vi "Leaderboard test 5.vi"(11 "current time":timestamp) -> ()   [LabVIEW 2020, in "Visualisation.lvclass"]
uses:
  Visualisation.lvclass
  Application/Globals.vi
  Data Manager/Data Manager.lvclass
  Application/Application.lvlib
panel:
  out "Daily Change B":dbl format="+ %0.1f km"
  out "Daily Change A":dbl format="+ %0.1f km"
  out "Table Control":string[][](table)
  out "Line 3":string
  out "Group Totals 6":dbl format="%0.1f km"
  out "Group Totals 5":dbl format="%0.1f km"
  out "Line 2":string
  out "Group Totals 4":dbl format="%0.1f km"
  out "Group Totals 3":dbl format="%0.1f km"
  out "Line 1":string
  out "Group Totals 2":dbl format="%0.1f km"
  out "Group Totals 1":dbl format="%0.1f km"
  out "Walk":T1(array[cluster]) {"Distance 2" scale=0.0..92.6965}
  out "Leaderboard":T2(array[cluster]) {"Distance" scale=0.0..167.7288}
  out "Ride":T3(array[cluster]) {"Distance 4" scale=0.0..76.5197}
  out "Run":T1(array[cluster]) {"Distance 2" scale=0.0..96.2213}
  out "B Total":dbl format="%0.1f km"
  out "A Total":dbl format="%0.1f km"
  # "Total Distance Leaderboard"
  # "Head to Head"
  # "VS"
  # "VS"
  # "VS"
  # "Longest Single Activity"
  # "Daily Total Distance Change"
  # "VS"
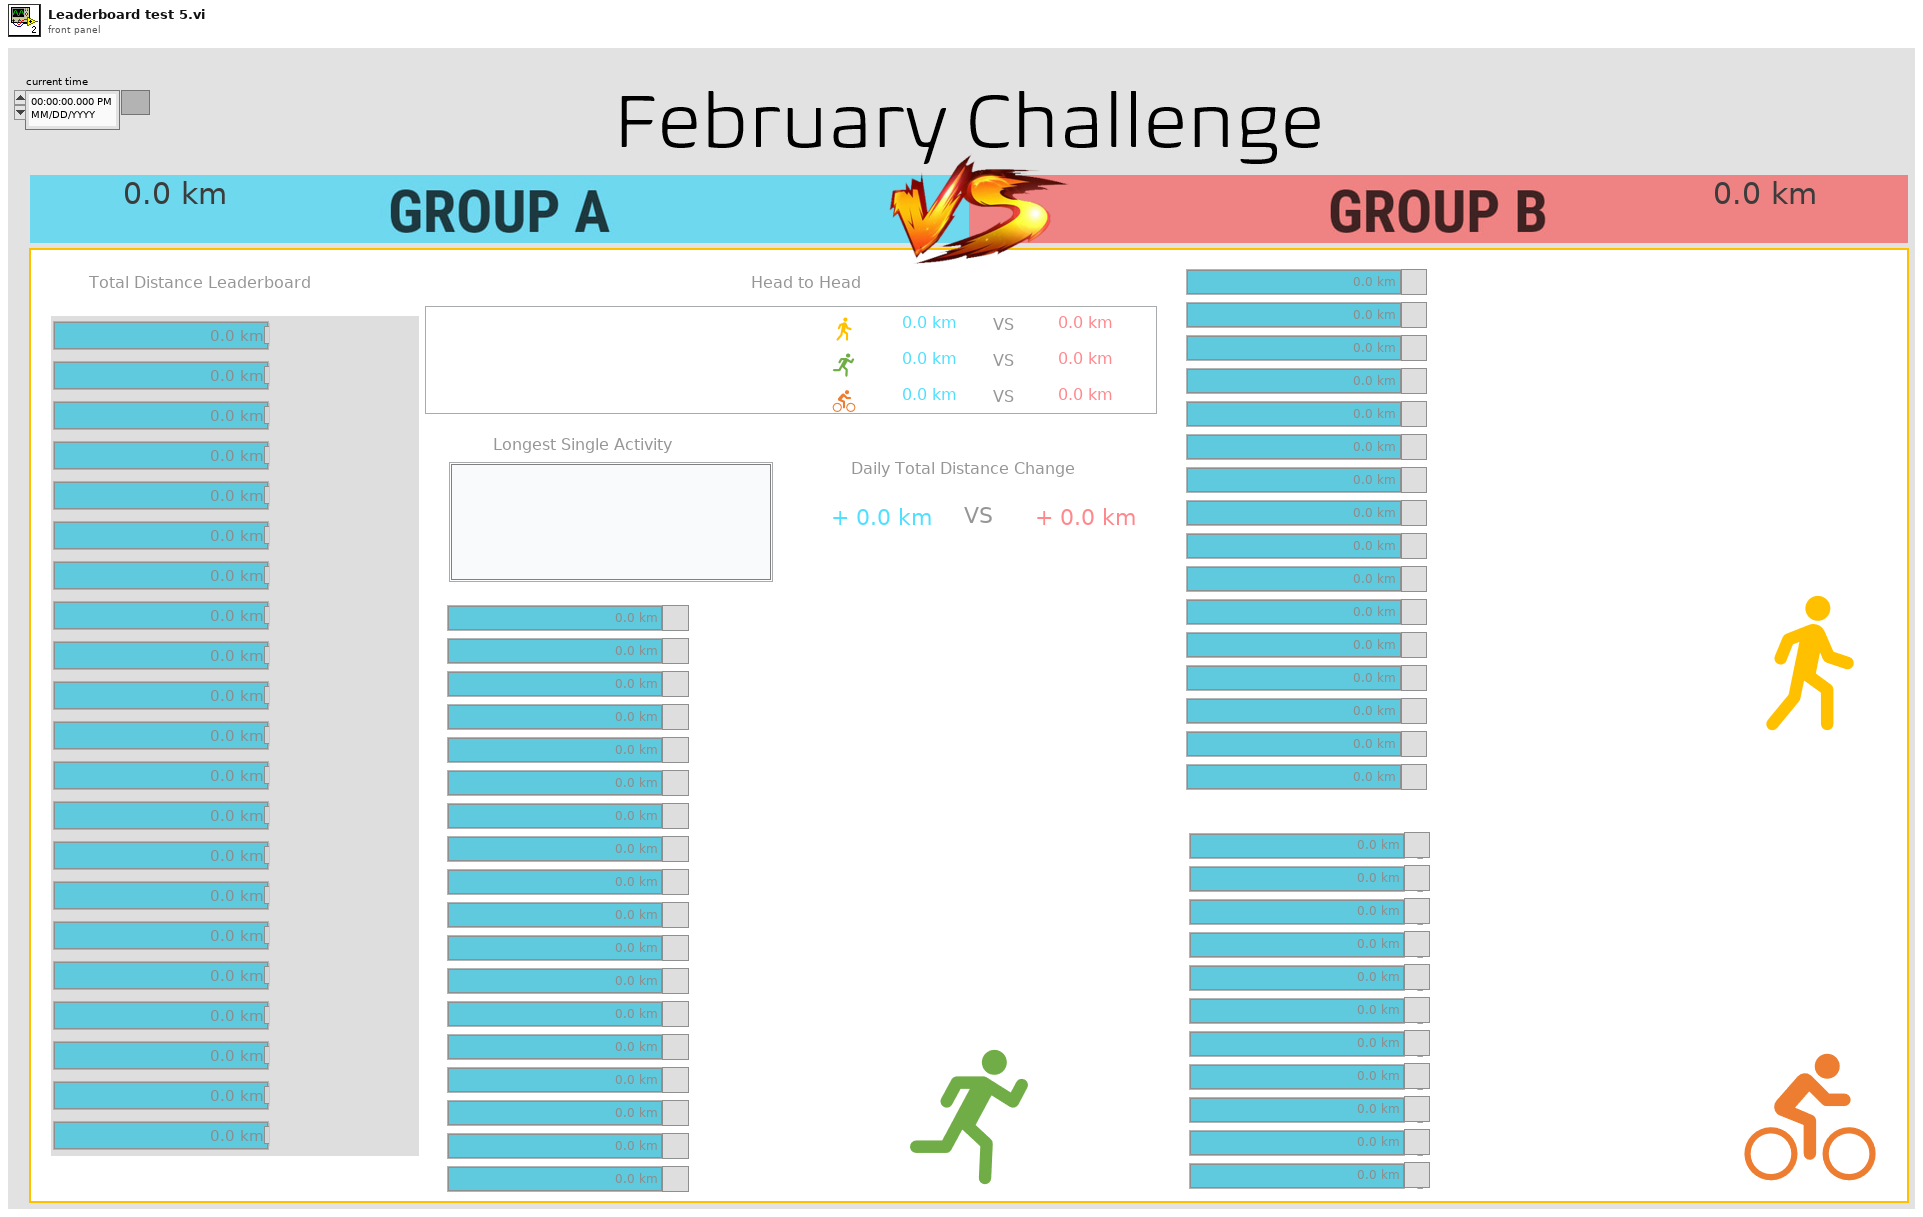
[diagram p1: front panel]
types:
  T1 = cluster{"Athlete":string, "Team":u32, "Distance 2":dbl}[]
  T2 = cluster{"Athlete":string, "Distance":dbl, "Team":u32}[]
  T3 = cluster{"Athlete":string, "Team":u32, "Distance 4":dbl}[]
  T4 = cluster{"Athlete":string, "Team":u32, "Distance 2":dbl}
  T5 = cluster{"Athlete":string, "Distance":dbl, "Team":u32, "Distance 2":cluster{"Numeric":dbl, "Numeric":dbl, "Numeric":dbl}}
  T6 = cluster{"Athlete":string, "Distance":dbl, "Team":u32}
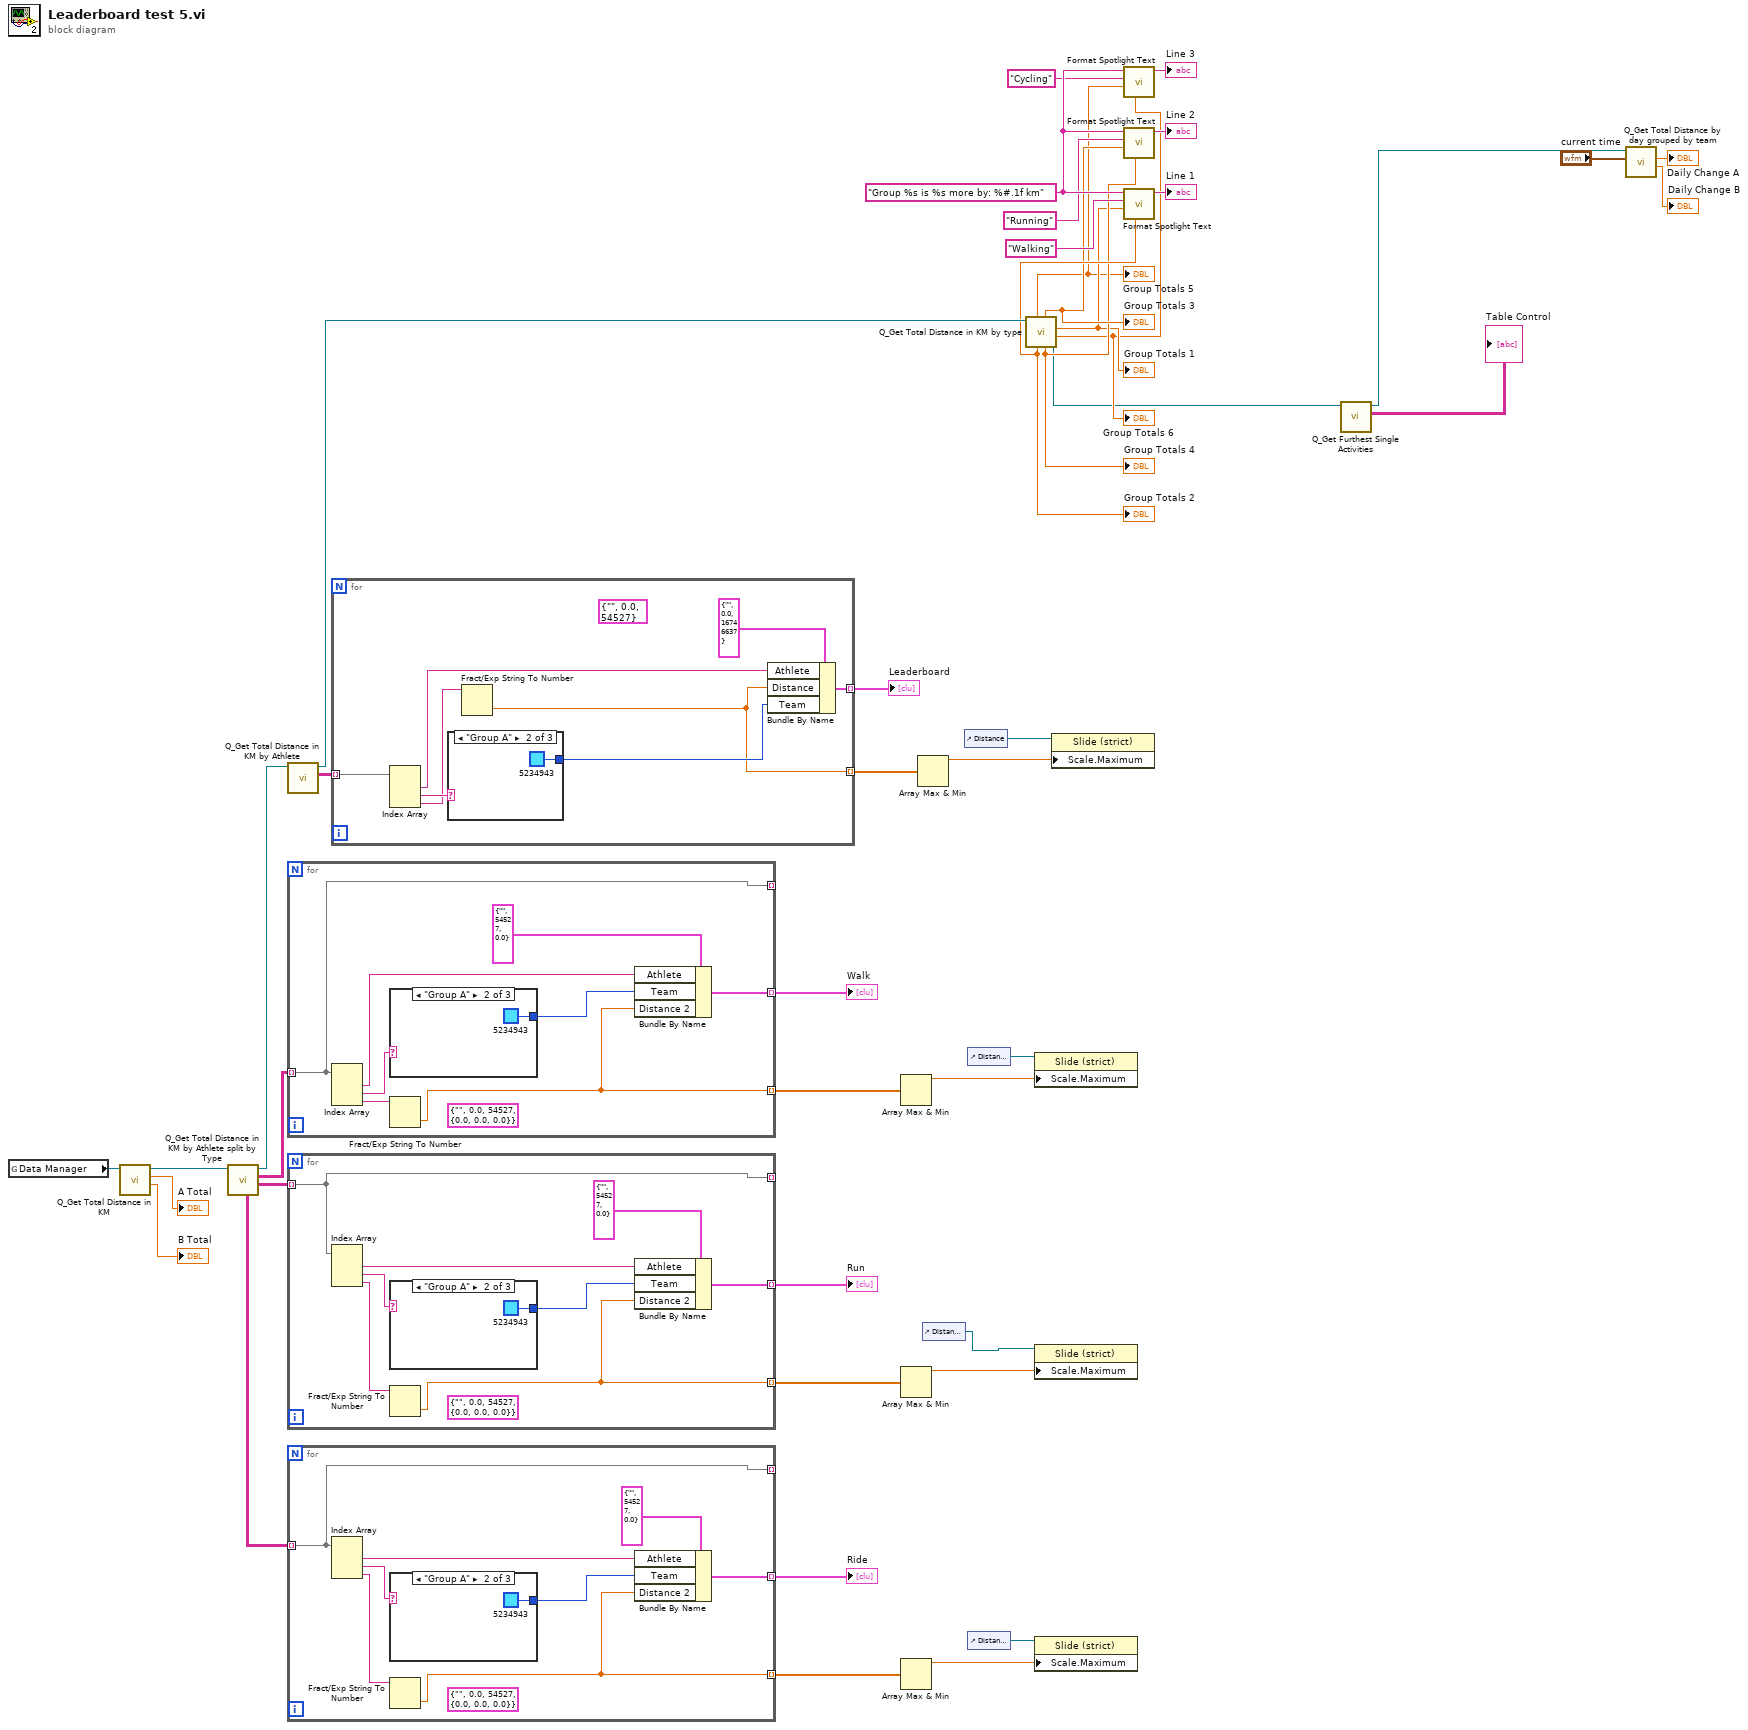
[diagram p0: block diagram]
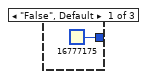
[diagram p2: hidden frame]
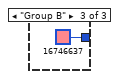
[diagram p3: hidden frame]
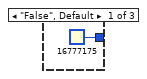
[diagram p4: hidden frame]
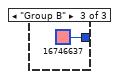
[diagram p5: hidden frame]
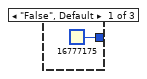
[diagram p6: hidden frame]
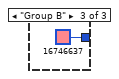
[diagram p7: hidden frame]
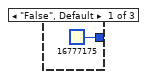
[diagram p8: hidden frame]
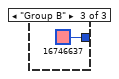
[diagram p9: hidden frame]
diagram:
  w16 = "Group %s is %s more by: %#.1f km"
  n1 = global read "Globals.vi" "Data Manager"() -> (w45:refnum<class "Data Manager.lvclass">)
  n2 = call-dynamic "Q_Get Total Distance in KM.vi"("Data Manager in"=w45) -> ("Group B"=→"B Total":dbl, "Group A"=→"A Total":dbl, "Data Manager out"=w40:refnum<class "Data Manager.lvclass">)  [unwired: 6 in, 2 out]
  n3 = call-dynamic "Q_Get Total Distance in KM by Athlete split by Type.vi"("Data Manager in"=w40) -> ("Run"=w35:string[][], "Walk"=w39:string[][], "Data Manager out"=w28:refnum<class "Data Manager.lvclass">, "Ride"=w32:string[][])  [unwired: 6 in, 1 out]
  n4 = call-dynamic "Q_Get Total Distance in KM by Athlete.vi"("Data Manager in"=w28) -> ("Result Set"=w27:string[][], "Data Manager out"=w20:refnum<class "Data Manager.lvclass">)  [unwired: 8 in, 1 out]
  n5 = for {
    tunnel: [w48] -> _ mode=indexing
    tunnel: [w53] -> w22 mode=indexing
    tunnel: w39 -> [w48] mode=indexing
    tunnel: [w47] -> w36 mode=indexing
    (unwired) T5 {"Athlete"="", "Distance"=0.0, "Team"=54527, "Distance 2"={"Numeric"=0.0, "Numeric"=0.0, "Numeric"=0.0}} ("Leaderboard")
    n6 = Index Array(array=w48) -> (element #1=w49:string, element #2=w51:string, element #3=w50:string)  [unwired: 3 in]
    n7 = case shown="\"Group A\"" w51 {
      tunnel: [u32 16777175 ("Color Box") u32 5234943 ("Color Box") u32 16746637 ("Color Box")] -> w52
      frame "False", Default {
      }
      frame "Group A" {
      }
      frame "Group B" {
      }
    }
    n8 = Fract/Exp String To Number(string=w50) -> (number=w47:dbl)  [unwired: 3 in, 1 out]
    n9 = Bundle By Name(cluster=T4 {"Athlete"="", "Team"=54527, "Distance 2"=0.0} ("Leaderboard"), "Athlete"=w49, "Team"=w52, "Distance 2"=w47) -> (w53:T4)
  }
  "Walk" <- w22
  n10 = for {
    tunnel: w35 -> [w59] mode=indexing
    tunnel: [w64] -> w33 mode=indexing
    tunnel: [w59] -> _ mode=indexing
    tunnel: [w58] -> w34 mode=indexing
    (unwired) T5 {"Athlete"="", "Distance"=0.0, "Team"=54527, "Distance 2"={"Numeric"=0.0, "Numeric"=0.0, "Numeric"=0.0}} ("Leaderboard")
    n11 = Index Array(array=w59) -> (element #1=w60:string, element #2=w62:string, element #3=w61:string)  [unwired: 3 in]
    n12 = case shown="\"Group A\"" w62 {
      tunnel: [u32 16777175 ("Color Box") u32 5234943 ("Color Box") u32 16746637 ("Color Box")] -> w63
      frame "False", Default {
      }
      frame "Group A" {
      }
      frame "Group B" {
      }
    }
    n13 = Fract/Exp String To Number(string=w61) -> (number=w58:dbl)  [unwired: 3 in, 1 out]
    n14 = Bundle By Name(cluster=T4 {"Athlete"="", "Team"=54527, "Distance 2"=0.0} ("Leaderboard"), "Athlete"=w60, "Team"=w63, "Distance 2"=w58) -> (w64:T4)
  }
  "Run" <- w33
  n15 = for {
    tunnel: w32 -> [w70] mode=indexing
    tunnel: [w75] -> w30 mode=indexing
    tunnel: [w70] -> _ mode=indexing
    tunnel: [w69] -> w31 mode=indexing
    (unwired) T5 {"Athlete"="", "Distance"=0.0, "Team"=54527, "Distance 2"={"Numeric"=0.0, "Numeric"=0.0, "Numeric"=0.0}} ("Leaderboard")
    n16 = Index Array(array=w70) -> (element #1=w71:string, element #2=w73:string, element #3=w72:string)  [unwired: 3 in]
    n17 = case shown="\"Group A\"" w73 {
      tunnel: [u32 16777175 ("Color Box") u32 5234943 ("Color Box") u32 16746637 ("Color Box")] -> w74
      frame "False", Default {
      }
      frame "Group A" {
      }
      frame "Group B" {
      }
    }
    n18 = Fract/Exp String To Number(string=w72) -> (number=w69:dbl)  [unwired: 3 in, 1 out]
    n19 = Bundle By Name(cluster=T4 {"Athlete"="", "Team"=54527, "Distance 2"=0.0} ("Leaderboard"), "Athlete"=w71, "Team"=w74, "Distance 2"=w69) -> (w75:T4)
  }
  "Ride" <- w30
  n20 = for {
    tunnel: w27 -> [w85] mode=indexing
    tunnel: [w86] -> w26 mode=indexing
    tunnel: [w79] -> w24 mode=indexing
    (unwired) T6 {"Athlete"="", "Distance"=0.0, "Team"=54527} ("Leaderboard")
    n21 = Index Array(array=w85) -> (element #1=w81:string, element #2=w83:string, element #3=w82:string)  [unwired: 3 in]
    n22 = case shown="\"Group A\"" w83 {
      tunnel: [u32 16777175 ("Color Box") u32 5234943 ("Color Box") u32 16746637 ("Color Box")] -> w84
      frame "False", Default {
      }
      frame "Group A" {
      }
      frame "Group B" {
      }
    }
    n23 = Fract/Exp String To Number(string=w82) -> (number=w79:dbl)  [unwired: 3 in, 1 out]
    n24 = Bundle By Name(cluster=T6 {"Athlete"="", "Distance"=0.0, "Team"=16746637} ("Leaderboard"), "Athlete"=w81, "Distance"=w79, "Team"=w84) -> (w86:T6)
  }
  "Leaderboard" <- w26
  n25 = Array Max & Min(array=w36) -> (max value=w37:dbl)  [unwired: 3 out]
  n26 = Array Max & Min(array=w34) -> (max value=w42:dbl)  [unwired: 3 out]
  n27 = Array Max & Min(array=w31) -> (max value=w41:dbl)  [unwired: 3 out]
  n28 = Array Max & Min(array=w24) -> (max value=w25:dbl)  [unwired: 3 out]
  n29 = control-ref of="Distance 2"() -> (w21:refnum<vi>)
  n30 = control-ref of="Distance"() -> (w23:refnum<vi>)
  n31 = control-ref of="Distance 2"() -> (w38:refnum<vi>)
  n32 = control-ref of="Distance 4"() -> (w29:refnum<vi>)
  n33 = call-dynamic "Q_Get Total Distance in KM by type.vi"("Data Manager in"=w20) -> ("B Ride"=w7:dbl, "A Walk"=w9:dbl, "Data Manager out"=w6:refnum<class "Data Manager.lvclass">, "Run"=w10:dbl, "A Run"=w11:dbl, "Walk"=w19:dbl, "A Ride"=w8:dbl)  [unwired: 3 in, 1 out]
  "Group Totals 1" <- w9
  "Group Totals 2" <- w19
  "Group Totals 3" <- w11
  "Group Totals 4" <- w10
  "Group Totals 5" <- w8
  "Group Totals 6" <- w7
  n34 = property on="Property Node" class="Slide (strict)"(reference=w38, "Scale.Maximum"=w37) -> ()  [unwired: 1 in, 2 out]
  n35 = property on="Property Node" class="Slide (strict)"(reference=w21, "Scale.Maximum"=w42) -> ()  [unwired: 1 in, 2 out]
  n36 = property on="Property Node" class="Slide (strict)"(reference=w29, "Scale.Maximum"=w41) -> ()  [unwired: 1 in, 2 out]
  n37 = property on="Property Node" class="Slide (strict)"(reference=w23, "Scale.Maximum"=w25) -> ()  [unwired: 1 in, 2 out]
  n38 = call "Format Spotlight Text.vi"("Walk"=w7, "A Walk"=w8, "String"="Cycling", "String 2"=w16) -> ("String 3"=→"Line 3":string)  [unwired: 7 in]
  n39 = call "Format Spotlight Text.vi"("Walk"=w10, "A Walk"=w11, "String"="Running", "String 2"=w16) -> ("String 3"=→"Line 2":string)  [unwired: 7 in]
  n40 = call "Format Spotlight Text.vi"("Walk"=w19, "A Walk"=w9, "String"="Walking", "String 2"=w16) -> ("String 3"=→"Line 1":string)  [unwired: 7 in]
  n41 = call-dynamic "Q_Get Furthest Single Activities.vi"("Data Manager in"=w6) -> ("Result Set"=→"Table Control":string[][], "Data Manager out"=w4:refnum<class "Data Manager.lvclass">)  [unwired: 8 in, 1 out]
  n42 = call-dynamic "Q_Get Total Distance by day grouped by team.vi"("current time"="current time", "Data Manager in"=w4) -> ("Group B Daily"=→"Daily Change B":dbl, "Group A Daily"=→"Daily Change A":dbl)  [unwired: 6 in, 2 out]
